vi "pp_sessList_isValid.vi"(0 "Trial Types":T1(array[cluster]) {"Stim P2" min=0.0; "Trial Weight" step=1; "Stim P1" min=0.0; "Stim Dur (s)" min=0.0; "Trial Code" min=1 step=1}, 5 "Total Trials":i32=60 min=2 step=2, 9 "Session List":i32[](array[numeric]), 13 "Trial Replication Factor":i32) -> (4 "Session List Valid?":bool=TRUE)   [LabVIEW 2013]
uses:
  labolabo/array/impl/ArrayRemove_I.vi
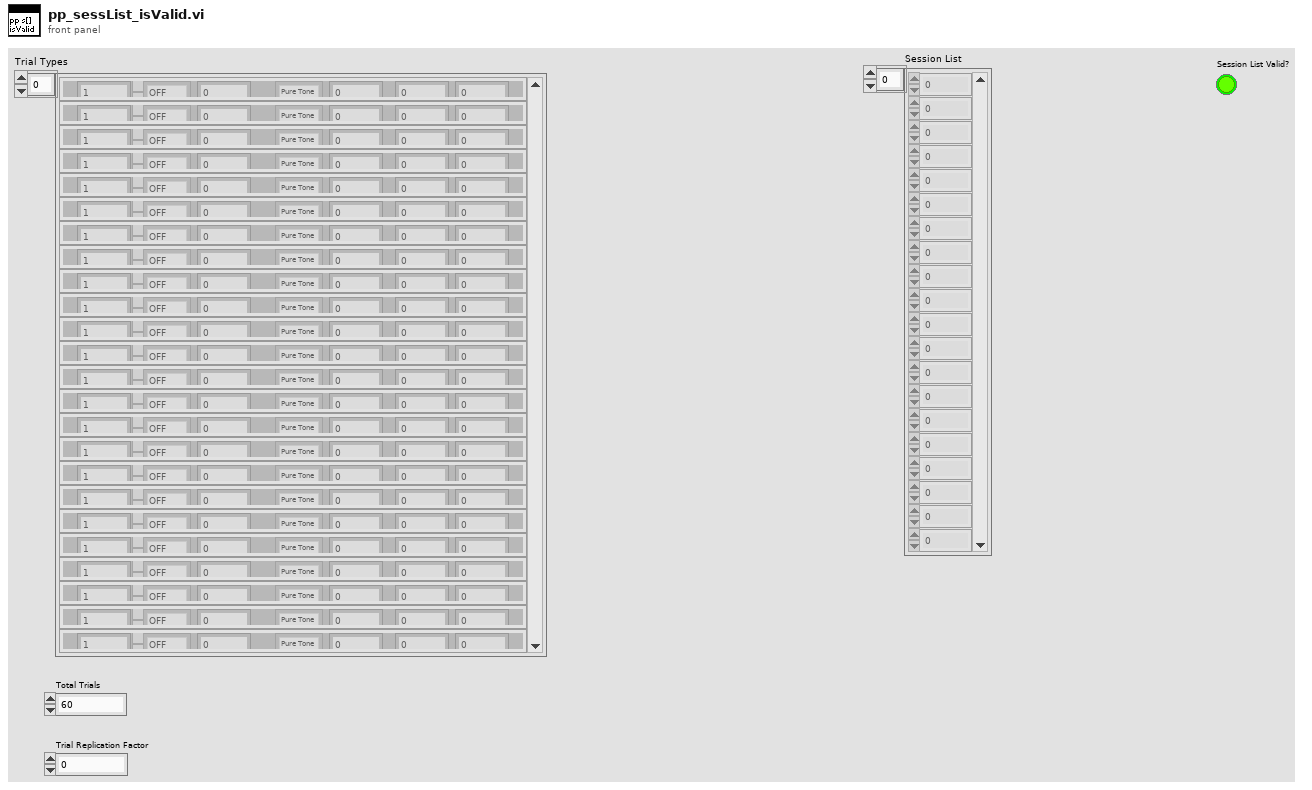
[diagram p1: front panel]
types:
  T1 = cluster{"Trial Code":u16, "Trial Type":enum16{"OFF", "GO", "NOGO", "TEST"}, "Trial Weight":u32, "Stim Type":enum16{"Pure Tone", "FM Sweep"}, "Stim Dur (s)":dbl, "Stim P1":dbl, "Stim P2":dbl}[]
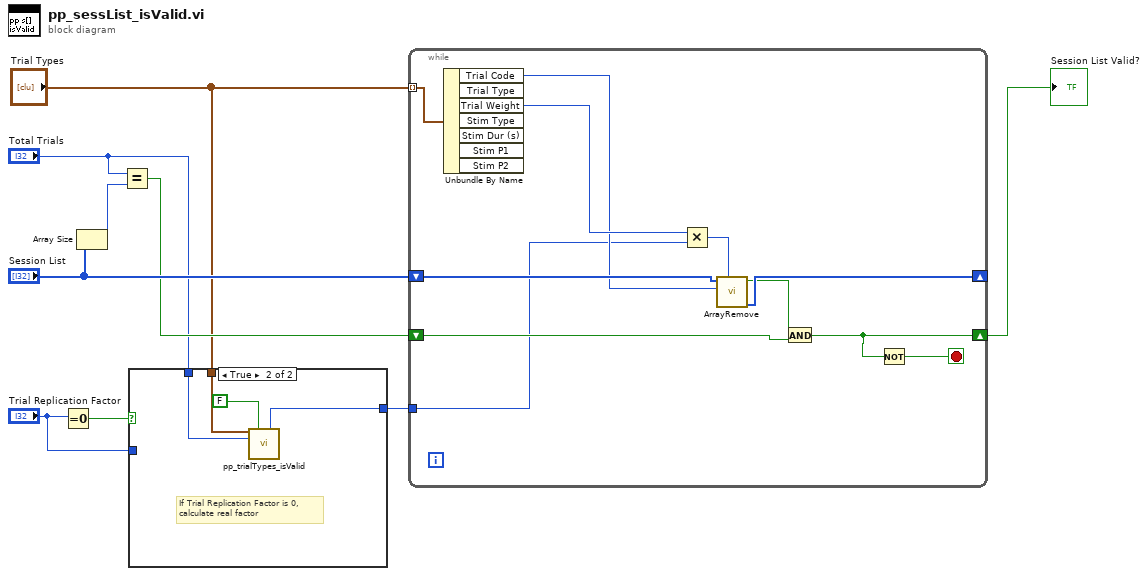
[diagram p0: block diagram]
diagram:
  n1 = Equal To 0?(x="Trial Replication Factor") -> (x = 0?=w5:bool)
  n2 = Array Size(array="Session List") -> (size(s)=w9:i32)
  n3 = Equal?(x="Total Trials", y=w9) -> (x = y?=w7:bool)
  n4 = case shown="True" w5 {
    tunnel: "Trial Replication Factor" -> [w10 _]
    tunnel: [w10 w14] -> w1
    tunnel: "Trial Types" -> [_ w13]
    tunnel: "Total Trials" -> [_ w12]
    frame False {
    }
    frame True {
      # "If Trial Replication Factor is 0,\ncalculate real factor"
      n5 = call "pp_trialTypes_isValid.vi"("Trial Types"=w13, "Throw Error"=FALSE, "Total Trials"=w12) -> ("Trial Replication Factor"=w14:i32)  [unwired: 7 in, 5 out]
    }
  }
  n6 = while {
    tunnel: "Trial Types" -> [w25] mode=indexing
    shift-right: [w23] -> _
    shift-left: "Session List" -> [w24]
    shift-right: [w17] -> w6
    shift-left: w7 -> [w21]
    tunnel: w1 -> [w15]
    stop <- w16 stop-if-true
    n7 = Unbundle By Name(w25) -> ("Trial Code"=w18:u16, "Trial Weight"=w20:u32)  [unwired: 5 out]
    n8 = Multiply(x=w20, y=w15) -> (x*y=w19:u32)
    n9 = call-poly "ArrayRemove.vi"("N"=w19, "To Remove"=w18, "1D Array In"=w24) -> ("1D Array Out"=w23:i32[], "Removed All"=w22:bool)  [unwired: 7 in]
    n10 = And(x=w22, y=w21) -> (x .and. y?=w17:bool)
    n11 = Not(x=w17) -> (.not. x?=w16:bool)
  }
  "Session List Valid?" <- w6
